vi "Arrange 2 Graph.vi"(4 "AngleMaxForce":bool, 5 "Find Fist Touch":bool, 6 "AngleUpDown":T1, 8 "Analog RW Up":T2, 9 "Analog FW Up":T2, 10 "Analog RW Down":T2, 11 "Analog FW Down":T2) -> (0 "Signal Up":T3, 3 "Signal Down":T4)   [LabVIEW 2017]
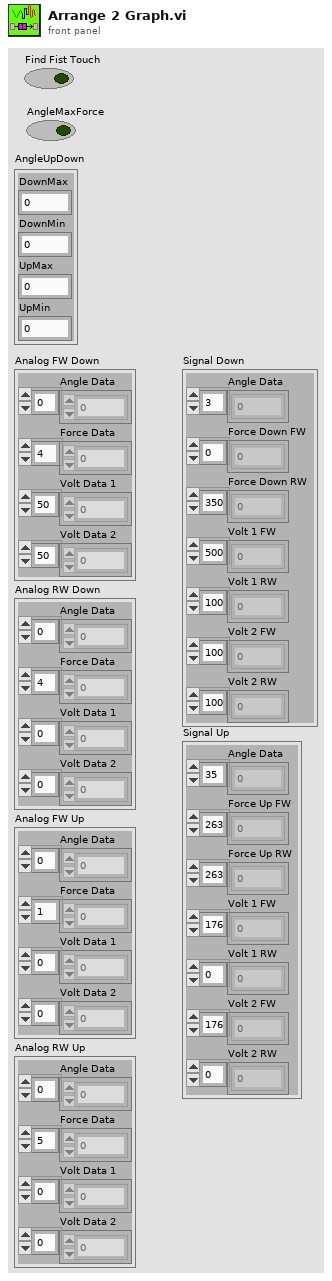
[diagram p1: front panel]
types:
  T1 = cluster{"DownMax":u16, "DownMin":u16, "UpMax":u16, "UpMin":u16}
  T2 = cluster{"Angle Data":dbl[], "Force Data":dbl[], "Volt Data 1":dbl[], "Volt Data 2":dbl[]}
  T3 = cluster{"Angle Data":dbl[], "Force Up FW":dbl[], "Force Up RW":dbl[], "Volt 1 FW":dbl[], "Volt 1 RW":dbl[], "Volt 2 FW":dbl[], "Volt 2 RW":dbl[]}
  T4 = cluster{"Angle Data":dbl[], "Force Down FW":dbl[], "Force Down RW":dbl[], "Volt 1 FW":dbl[], "Volt 1 RW":dbl[], "Volt 2 FW":dbl[], "Volt 2 RW":dbl[]}
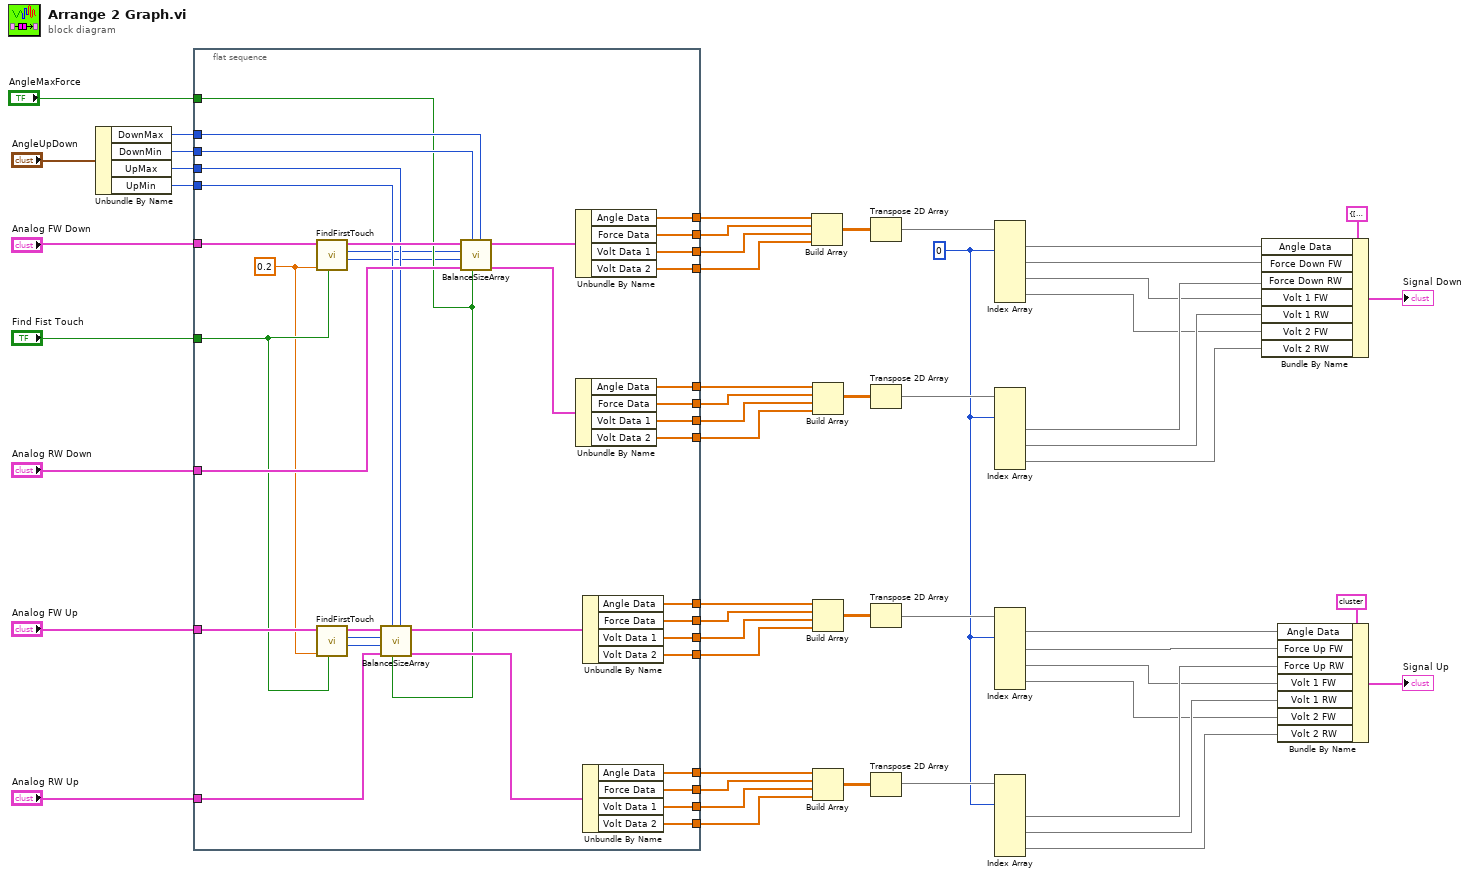
[diagram p0: block diagram]
diagram:
  w3 = 0 ("disabled index (col)")
  n1 = Unbundle By Name("AngleUpDown") -> ("DownMax"=w33:u16, "DownMin"=w32:u16, "UpMax"=w27:u16, "UpMin"=w26:u16)
  n2 = flat-sequence {
    tunnel: [w80] -> w1
    tunnel: [w81] -> w43
    tunnel: [w82] -> w42
    tunnel: [w83] -> w44
    tunnel: [w84] -> w45
    tunnel: [w85] -> w2
    tunnel: [w86] -> w8
    tunnel: [w87] -> w47
    tunnel: [w88] -> w46
    tunnel: [w89] -> w48
    tunnel: [w90] -> w49
    tunnel: [w91] -> w50
    tunnel: "Analog FW Down" -> [w72]
    tunnel: "Analog RW Down" -> [w78]
    tunnel: "Analog FW Up" -> [w73]
    tunnel: "Analog RW Up" -> [w75]
    tunnel: "Find Fist Touch" -> [w71]
    tunnel: w33 -> [w62]
    tunnel: w32 -> [w63]
    tunnel: w27 -> [w60]
    tunnel: w26 -> [w61]
    tunnel: "AngleMaxForce" -> [w59]
    tunnel: [w67] -> w10
    tunnel: [w66] -> w9
    tunnel: [w65] -> w7
    tunnel: [w64] -> w6
    frame #0 {
      w70 = 0.2 ("Level Reference")
      n3 = call "FindFirstTouch.vi"("EN"=w71, "Level Reference"=w70, "Analog FW In"=w72) -> ("CounterDeleteOut"=w57:i32, "TotalSizeOut"=w58:i32, "Analog FW Out"=w79:T2)  [unwired: 6 in]
      n4 = call "FindFirstTouch.vi"("EN"=w71, "Level Reference"=w70, "Analog FW In"=w73) -> ("CounterDeleteOut"=w55:i32, "TotalSizeOut"=w56:i32, "Analog FW Out"=w76:T2)  [unwired: 6 in]
      n5 = call "BalanceSizeArray.vi"("Max Stroke"=w60, "MaxForce"=w59, "Min Stroke"=w61, "Analog RW In"=w75, "CountDeleteIn"=w55, "TotalSizeIn"=w56, "Analog FW In"=w76) -> ("Analog RW Out"=w74:T2, "Analog FW Out"=w68:T2)  [unwired: 3 in]
      n6 = call "BalanceSizeArray.vi"("Max Stroke"=w62, "MaxForce"=w59, "Min Stroke"=w63, "Analog RW In"=w78, "CountDeleteIn"=w57, "TotalSizeIn"=w58, "Analog FW In"=w79) -> ("Analog RW Out"=w77:T2, "Analog FW Out"=w69:T2)  [unwired: 3 in]
      n7 = Unbundle By Name(w69) -> ("Angle Data"=w67:dbl[], "Force Data"=w91:dbl[], "Volt Data 1"=w90:dbl[], "Volt Data 2"=w89:dbl[])
      n8 = Unbundle By Name(w77) -> ("Angle Data"=w66:dbl[], "Force Data"=w86:dbl[], "Volt Data 1"=w87:dbl[], "Volt Data 2"=w88:dbl[])
      n9 = Unbundle By Name(w68) -> ("Angle Data"=w65:dbl[], "Force Data"=w85:dbl[], "Volt Data 1"=w84:dbl[], "Volt Data 2"=w83:dbl[])
      n10 = Unbundle By Name(w74) -> ("Angle Data"=w64:dbl[], "Force Data"=w80:dbl[], "Volt Data 1"=w81:dbl[], "Volt Data 2"=w82:dbl[])
    }
  }
  n11 = Build Array(w10, w50, w49, w48) -> (w41:dbl[][])
  n12 = Build Array(w9, w8, w47, w46) -> (w38:dbl[][])
  n13 = Build Array(w7, w2, w45, w44) -> (w39:dbl[][])
  n14 = Build Array(w6, w1, w43, w42) -> (w36:dbl[][])
  n15 = Transpose 2D Array(2D array=w41) -> (transposed array=w40:dbl[][])
  n16 = Transpose 2D Array(2D array=w38) -> (transposed array=w37:dbl[][])
  n17 = Transpose 2D Array(2D array=w39) -> (transposed array=w15:dbl[][])
  n18 = Transpose 2D Array(2D array=w36) -> (transposed array=w14:dbl[][])
  n19 = Index Array(array=w40, index (col) #1=w3) -> (element #1=w5:dbl[], element #2=w31:dbl[], element #3=w28:dbl[], element #4=w23:dbl[])  [unwired: 7 in]
  n20 = Index Array(array=w37, index (col) #1=w3) -> (element #2=w29:dbl[], element #3=w30:dbl[], element #4=w22:dbl[])  [unwired: 7 in, 1 out]
  n21 = Index Array(array=w15, index (col) #1=w3) -> (element #1=w4:dbl[], element #2=w21:dbl[], element #3=w19:dbl[], element #4=w17:dbl[])  [unwired: 7 in]
  n22 = Index Array(array=w14, index (col) #1=w3) -> (element #2=w20:dbl[], element #3=w18:dbl[], element #4=w16:dbl[])  [unwired: 7 in, 1 out]
  n23 = Bundle By Name(cluster=T4 {"Angle Data"=[], "Force Down FW"=[], "Force Down RW"=[], "Volt 1 FW"=[], "Volt 1 RW"=[], "Volt 2 FW"=[], "Volt 2 RW"=[]} ("Signal Down Data"), "Angle Data"=w5, "Force Down FW"=w31, "Force Down RW"=w29, "Volt 1 FW"=w28, "Volt 1 RW"=w30, "Volt 2 FW"=w23, "Volt 2 RW"=w22) -> (→"Signal Down":T4)
  n24 = Bundle By Name(cluster=T3 {"Angle Data"=array[513 elements], "Force Up FW"=array[562 elements], "Force Up RW"=array[562 elements], "Volt 1 FW"=array[562 elements], "Volt 1 RW"=array[562 elements], "Volt 2 FW"=array[562 elements], "Volt 2 RW"=array[562 elements]} ("Signal Up Data"), "Angle Data"=w4, "Force Up FW"=w21, "Force Up RW"=w20, "Volt 1 FW"=w19, "Volt 1 RW"=w18, "Volt 2 FW"=w17, "Volt 2 RW"=w16) -> (→"Signal Up":T3)
